vi "PC_Display.vi"() -> ()   [LabVIEW 2011]
panel:
  out "z out":sgl
  out "Waveform Chart":u32(graph)
  out "Derived":cluster{dbl, dbl}(graph)
  out "Command":cluster{dbl, dbl}(graph)
  out "Speed":cluster{dbl, dbl, dbl}(graph)
  in  "LinkRT":bool
  in  "Stop":bool
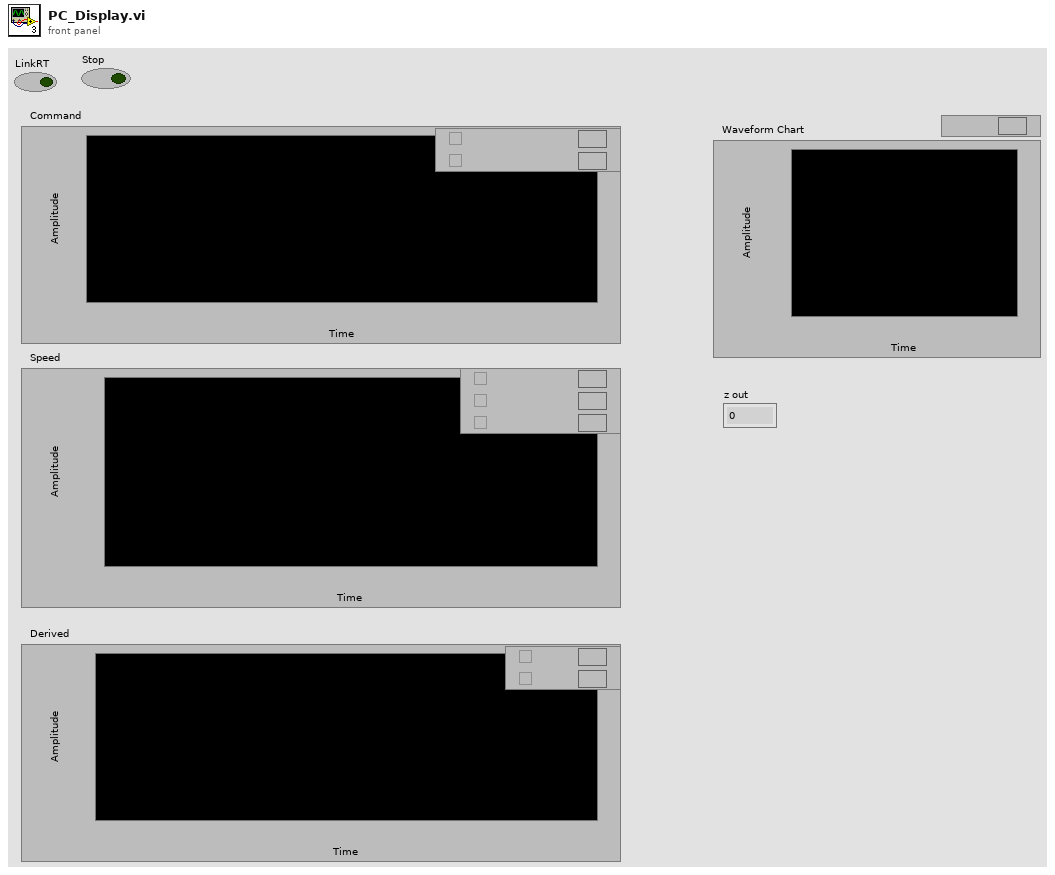
[diagram p1: front panel]
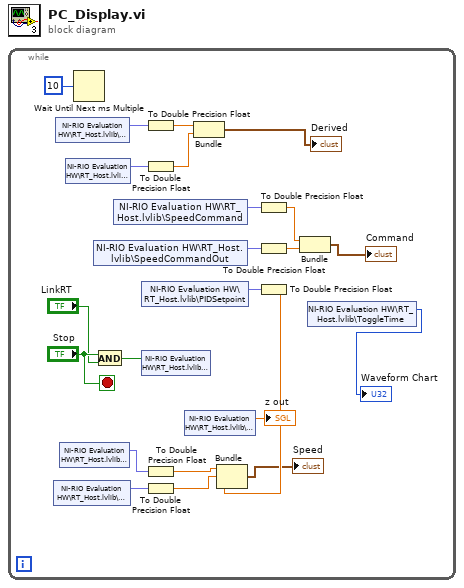
[diagram p0: block diagram]
diagram:
  n1 = while {
    stop <- "Stop" stop-if-true
    n2 = shared-variable "NI-RIO Evaluation HW\\RT_Host.lvlib\\Speed"() -> (w20:fxp<+/-,33,18>)  [unwired: 1 in, 1 out]
    n3 = shared-variable "NI-RIO Evaluation HW\\RT_Host.lvlib\\Accel"() -> (w19:fxp<+/-,33,18>)  [unwired: 1 in, 1 out]
    n4 = shared-variable "NI-RIO Evaluation HW\\RT_Host.lvlib\\RPM"() -> (w21:fxp<+,32,16>)  [unwired: 1 in, 1 out]
    n5 = shared-variable "NI-RIO Evaluation HW\\RT_Host.lvlib\\Jerk"() -> (w18:fxp<+/-,37,22>)  [unwired: 1 in, 1 out]
    n6 = Wait Until Next ms Multiple(millisecond multiple=u32 10) -> ()  [unwired: 1 out]
    n7 = shared-variable "NI-RIO Evaluation HW\\RT_Host.lvlib\\SpeedCommandOut"() -> (w11:fxp<+/-,23,8>)  [unwired: 1 in, 1 out]
    n8 = And(x="Stop", y="LinkRT") -> (x .and. y?=w17:bool)
    n9 = shared-variable "NI-RIO Evaluation HW\\RT_Host.lvlib\\SpeedCommand"() -> (w22:fxp<+/-,20,5>)  [unwired: 1 in, 1 out]
    n10 = shared-variable "NI-RIO Evaluation HW\\RT_Host.lvlib\\PIDSetpoint"() -> (w14:fxp<+/-,16,18>)  [unwired: 1 in, 1 out]
    n11 = shared-variable "NI-RIO Evaluation HW\\RT_Host.lvlib\\Stop"(w17) -> ()  [unwired: 1 in, 1 out]
    n12 = To Double Precision Float(number=w19) -> (double precision float=w13:dbl)
    n13 = To Double Precision Float(number=w18) -> (double precision float=w12:dbl)
    n14 = To Double Precision Float(number=w21) -> (double precision float=w8:dbl)
    n15 = To Double Precision Float(number=w20) -> (double precision float=w7:dbl)
    n16 = shared-variable "NI-RIO Evaluation HW\\RT_Host.lvlib\\z out"() -> (→"z out":sgl)  [unwired: 1 in, 1 out]
    n17 = Bundle(w13, w12) -> (→"Derived":cluster{dbl, dbl})  [unwired: 1 in]
    n18 = To Double Precision Float(number=w22) -> (double precision float=w10:dbl)
    n19 = To Double Precision Float(number=w11) -> (double precision float=w9:dbl)
    n20 = To Double Precision Float(number=w14) -> (double precision float=w4:dbl)
    n21 = Bundle(w8, w7, w4) -> (→"Speed":cluster{dbl, dbl, dbl})  [unwired: 1 in]
    n22 = Bundle(w10, w9) -> (→"Command":cluster{dbl, dbl})  [unwired: 1 in]
    n23 = shared-variable "NI-RIO Evaluation HW\\RT_Host.lvlib\\ToggleTime"() -> (→"Waveform Chart":u32)  [unwired: 1 in, 1 out]
  }
